vi "CtrlUtil.ShowHide Tab Page.vi"(2 "Show":bool, 3 "Tab Name":string="Maint", 4 "Tab Control":refnum<vi>) -> ()   [LabVIEW 2024, in "EQMF.lvlib" / "Controls.lvlib"]
uses:
  Controls.lvlib
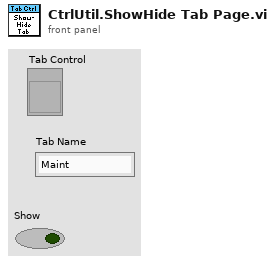
[diagram p1: front panel]
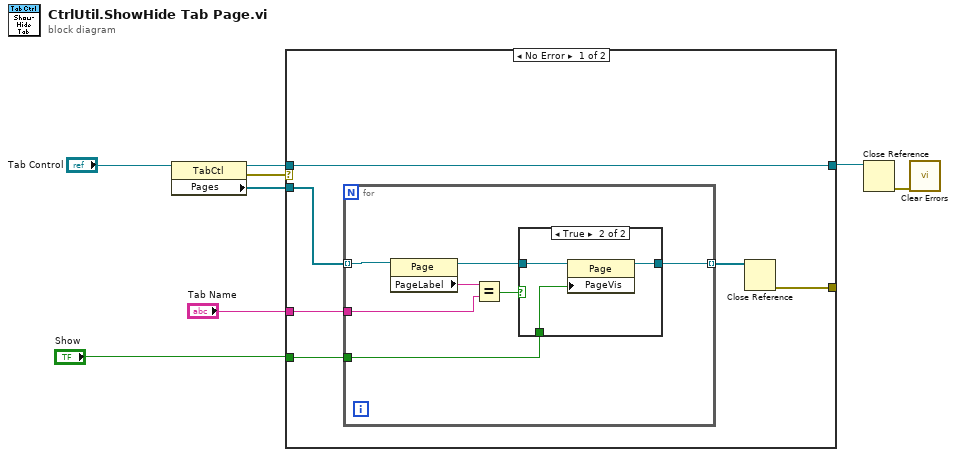
[diagram p0: block diagram]
diagram:
  n1 = property class="TabCtl"(reference="Tab Control") -> (reference out=w6:refnum<vi>, error out=w7:errorcluster, "Pages"=w8:refnum<vi>[])  [unwired: 1 in]
  n2 = case shown="No Error" w7 {
    tunnel: w8 -> [w14 _]
    tunnel: w6 -> [w13 w26]
    tunnel: [w13 w26] -> w5
    tunnel: [w11 _] -> _
    tunnel: "Show" -> [w10 _]
    tunnel: "Tab Name" -> [w9 _]
    frame No Error {
      n3 = for {
        tunnel: w14 -> [w21] mode=indexing
        tunnel: [w17] -> w12 mode=indexing
        tunnel: w10 -> [w16]
        tunnel: w9 -> [w15]
        n4 = property class="Page"(reference=w21) -> (reference out=w19:refnum<vi>, "PageLabel"=w20:string)  [unwired: 1 in, 1 out]
        n5 = Equal?(x=w20, y=w15) -> (x = y?=w18:bool)
        n6 = case shown="True" w18 {
          tunnel: w19 -> [w22 w25]
          tunnel: [w22 w24] -> w17
          tunnel: w16 -> [_ w23]
          frame False {
          }
          frame True {
            n7 = property class="Page"(reference=w25, "PageVis"=w23) -> (reference out=w24:refnum<vi>)  [unwired: 1 in, 1 out]
          }
        }
      }
      n8 = Close Reference(reference=w12) -> (error out=w11:errorcluster)  [unwired: 1 in]
    }
    frame Error {
      # "Do Nothing"
    }
  }
  n9 = Close Reference(reference=w5) -> (error out=w4:errorcluster)  [unwired: 1 in]
  n10 = call <vilib>:"Clear Errors.vi"("error in (no error)"=w4) -> ()  [unwired: 5 in, 2 out]
